vi "Check Rate.vi"(8 "amps?":bool, 9 "ramp":enum16{"Train Speed", "Maximum Speed", "Manual"}(ring), 10 "rate":dbl, 11 "field":dbl) -> (1 "maxrate":dbl, 2 "rateok":bool, 3 "rateOUT":dbl)   [LabVIEW 2009, in "Magnet.lvclass"]
uses:
  Magnet.lvclass
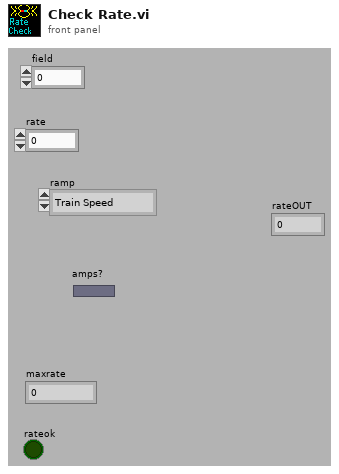
[diagram p1: front panel]
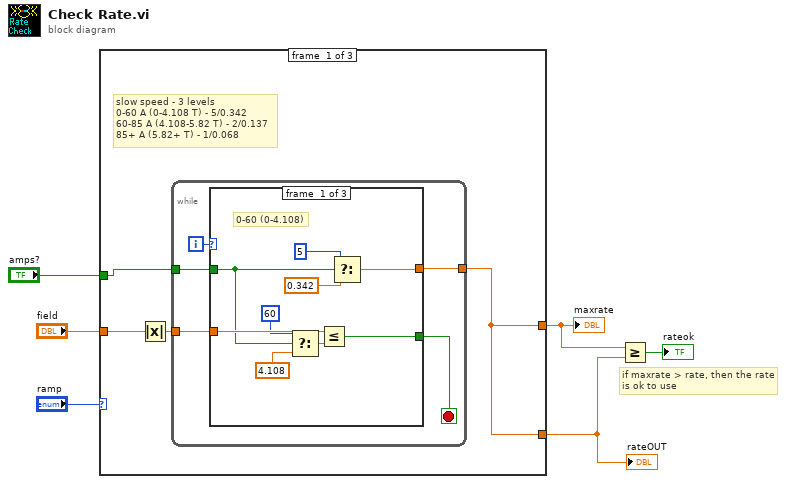
[diagram p0: block diagram]
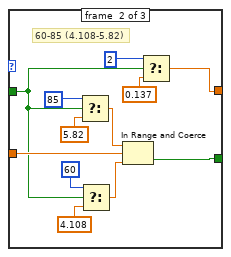
[diagram p2: hidden frame]
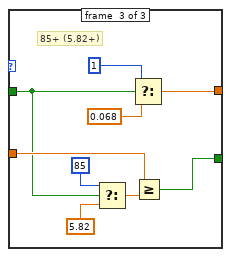
[diagram p3: hidden frame]
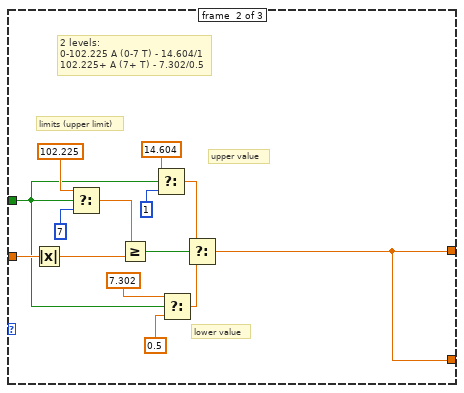
[diagram p4: hidden frame]
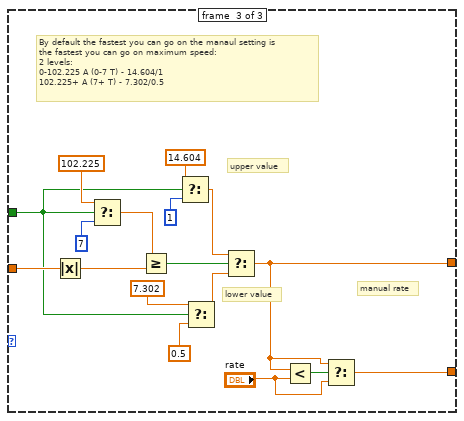
[diagram p5: hidden frame]
diagram:
  # "if maxrate > rate, then the rate\nis ok to use"
  n1 = case shown="\"Manual\"" "ramp" {
    tunnel: "field" -> [w10 w59 w71]
    tunnel: "amps?" -> [w8 w47 w64]
    tunnel: [w7 w46 w61] -> w3
    tunnel: [w7 w46 w60] -> w1
    frame #0 {
      # "slow speed - 3 levels\n0-60 A (0-4.108 T) - 5/0.342\n60-85 A (4.108-5.82 T) - 2/0.137\n85+ A (5.82+ T) - 1/0.068"
      n2 = Absolute Value(x=w10) -> (abs(x)=w9:dbl)
      n3 = while {
        tunnel: w9 -> [w14]
        tunnel: w8 -> [w12]
        tunnel: [w11] -> w7
        i -> [w15]
        stop <- w13 stop-if-true
        n4 = case shown="0, Default" w15 {
          tunnel: w14 -> [w24 w33 w42]
          tunnel: [w20 w30 w41] -> w13
          tunnel: w12 -> [w16 w25 w37]
          tunnel: [w17 w26 w38] -> w11
          frame #0 {
            # "0-60 (0-4.108)"
            n5 = Select(t=60, s=w16, f=4.108) -> (s? t:f=w21:dbl)
            n6 = Less Or Equal?(x=w24, y=w21) -> (x <= y?=w20:bool)
            n7 = Select(t=5, s=w16, f=0.342) -> (s? t:f=w17:dbl)
          }
          frame #1 {
            # "60-85 (4.108-5.82)"
            n8 = Select(t=85, s=w25, f=5.82) -> (s? t:f=w29:dbl)
            n9 = Select(t=60, s=w25, f=4.108) -> (s? t:f=w34:dbl)
            n10 = In Range and Coerce(upper limit=w29, x=w33, lower limit=w34) -> (In Range?=w30:bool)  [unwired: 1 out]
            n11 = Select(t=2, s=w25, f=0.137) -> (s? t:f=w26:dbl)
          }
          frame #2 {
            # "85+ (5.82+)"
            n12 = Select(t=85, s=w37, f=5.82) -> (s? t:f=w43:dbl)
            n13 = Select(t=1, s=w37, f=0.068) -> (s? t:f=w38:dbl)
            n14 = Greater Or Equal?(x=w42, y=w43) -> (x >= y?=w41:bool)
          }
        }
      }
    }
    frame #1 {
      # "limits (upper limit)"
      # "lower value"
      # "upper value"
      # "2 levels:\n0-102.225 A (0-7 T) - 14.604/1\n102.225+ A (7+ T) - 7.302/0.5"
      n15 = Absolute Value(x=w59) -> (abs(x)=w58:dbl)
      n16 = Select(t=102.225, s=w47, f=7) -> (s? t:f=w57:dbl)
      n17 = Greater Or Equal?(x=w57, y=w58) -> (x >= y?=w54:bool)
      n18 = Select(t=14.604, s=w47, f=1) -> (s? t:f=w51:dbl)
      n19 = Select(t=7.302, s=w47, f=0.5) -> (s? t:f=w48:dbl)
      n20 = Select(t=w51, s=w54, f=w48) -> (s? t:f=w46:dbl)
    }
    frame #2 {
      # "manual rate"
      # "lower value"
      # "upper value"
      # "By default the fastest you can go on the manaul setting is\nthe fastest you can go on maximum speed:\n2 levels:\n0-102.225 A (0-7 T) - 14.604/1\n102.225+ A (7+ T) - 7.302/0.5"
      n21 = Absolute Value(x=w71) -> (abs(x)=w76:dbl)
      n22 = Select(t=102.225, s=w64, f=7) -> (s? t:f=w75:dbl)
      n23 = Greater Or Equal?(x=w75, y=w76) -> (x >= y?=w72:bool)
      n24 = Select(t=14.604, s=w64, f=1) -> (s? t:f=w66:dbl)
      n25 = Select(t=7.302, s=w64, f=0.5) -> (s? t:f=w65:dbl)
      n26 = Select(t=w66, s=w72, f=w65) -> (s? t:f=w61:dbl)
      n27 = Less?(x=w61, y="rate") -> (x < y?=w63:bool)
      n28 = Select(t=w61, s=w63, f="rate") -> (s? t:f=w60:dbl)
    }
  }
  "maxrate" <- w3
  "rateOUT" <- w1
  n29 = Greater Or Equal?(x=w3, y=w1) -> (x >= y?=→"rateok":bool)
